vi "3.8.1.vi"() -> ()   [LabVIEW 2018]
panel:
  in  "열거형":enum16{"봄", "여름", "가을", "겨울"}(ring)
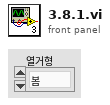
[diagram p1: front panel]
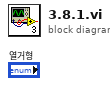
[diagram p0: block diagram]
diagram:
